vi "串口调试(hostlink).vi"(8 "error in (no error)":errorcluster caption="错误输入（无错误）", 11 "串口设置":T1={"VISA resource name"="COM1", "波特率"=9600, "数据位"=7, "停止位"=20, "奇偶位"=enum."Even"} {"停止位" items=["1.0"=10, "1.5"=15, "2.0"=20]; "数据位" items=["5"=5, "6"=6, "7"=7, "8"=8]; "波特率" items=["110"=110, "300"=300, "600"=600, "1200"=1200, "2400"=2400, "4800"=4800, "9600"=9600, "14400"=14400, "19200"=19200, "38400"=38400, "56000"=56000, "57600"=57600, "115200"=115200, "128000"=128000, "256000"=256000]}) -> (0 "error out":errorcluster caption="错误输出", 2 "串口状态":bool, 3 "串口初始化":T1)   [LabVIEW 2012]
uses:
  <vilib>/Instr/_visa.llb/VISA Flush IO Buffer Mask.ctl
  <vilib>/Instr/_visa.llb/VISA Configure Serial Port (Instr).vi
panel:
  out "返回码":string
  out "操作信息":string
  out "字符串接收区":string
  in  "过程停止按钮":bool
  in  "字符串发送区":string
  in  "发送":bool
  in  "取消按钮":bool
  in  "确定按钮":bool
  # "串口调试"
  # "(Omron Plc Hostlink 协议)"
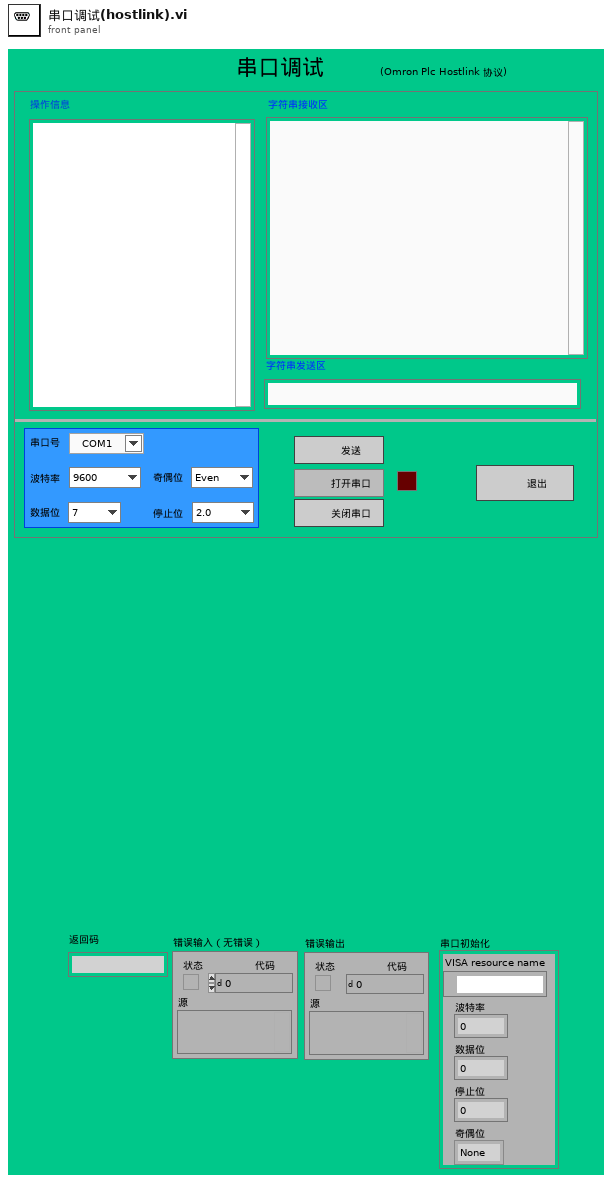
[diagram p1: front panel]
types:
  T1 = cluster{"VISA resource name":refnum<visa-resource-name>, "波特率":u32, "数据位":u16, "停止位":u16, "奇偶位":enum16{"None", "Odd", "Even", "Mark", "Space"}}
  T2 = typedef "VISA Flush IO Buffer Mask.ctl" = u16
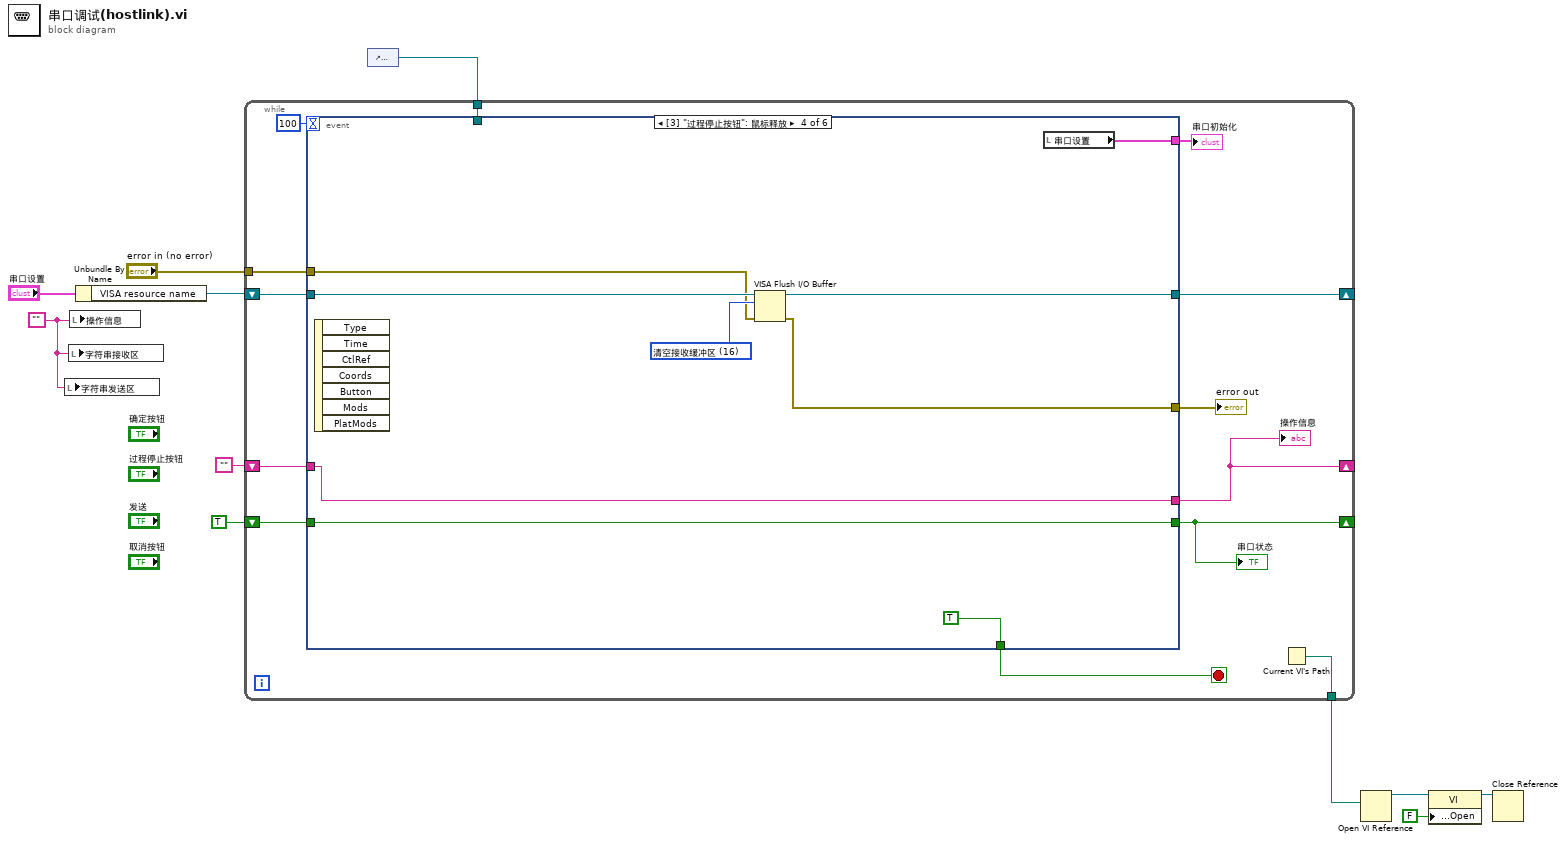
[diagram p0: block diagram]
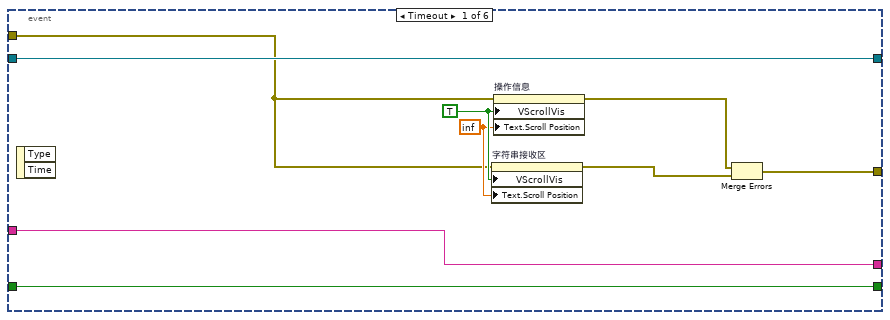
[diagram p2: hidden frame]
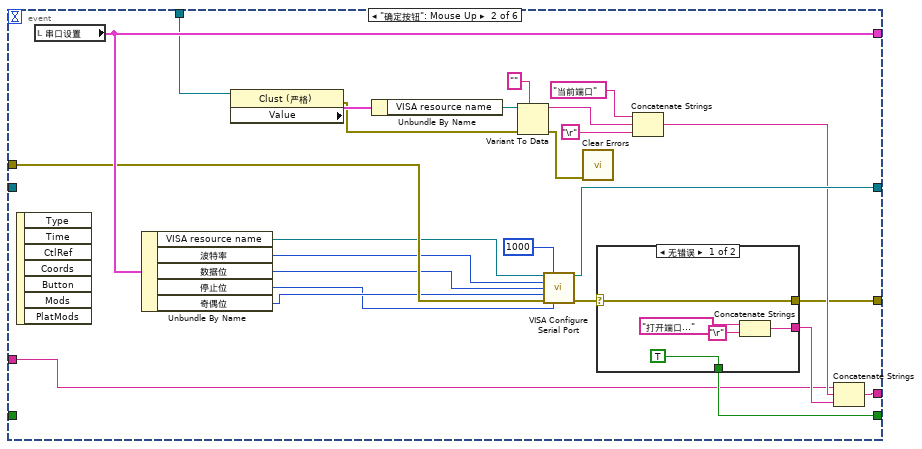
[diagram p3: hidden frame]
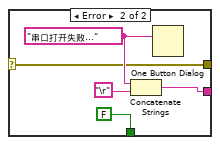
[diagram p4: hidden frame]
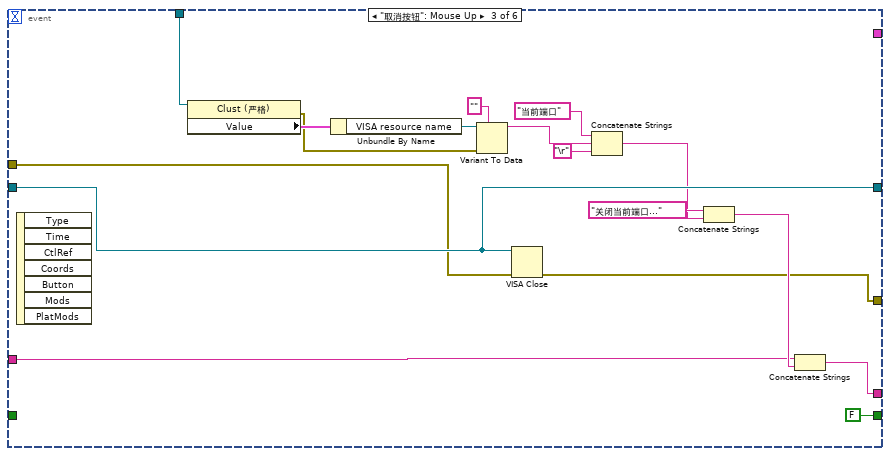
[diagram p5: hidden frame]
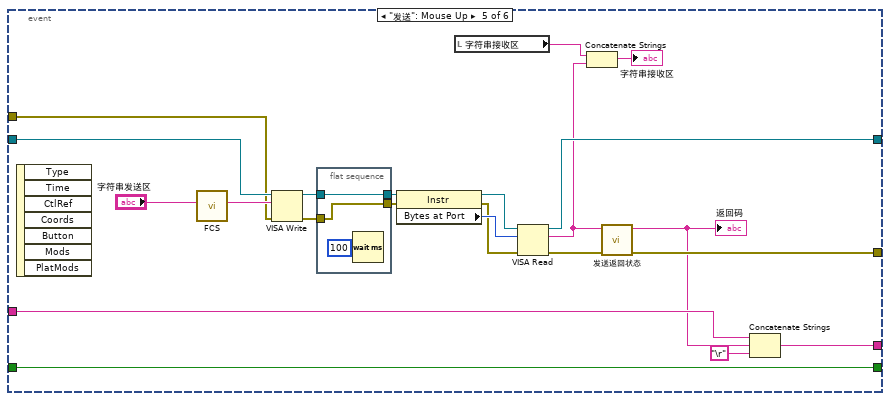
[diagram p6: hidden frame]
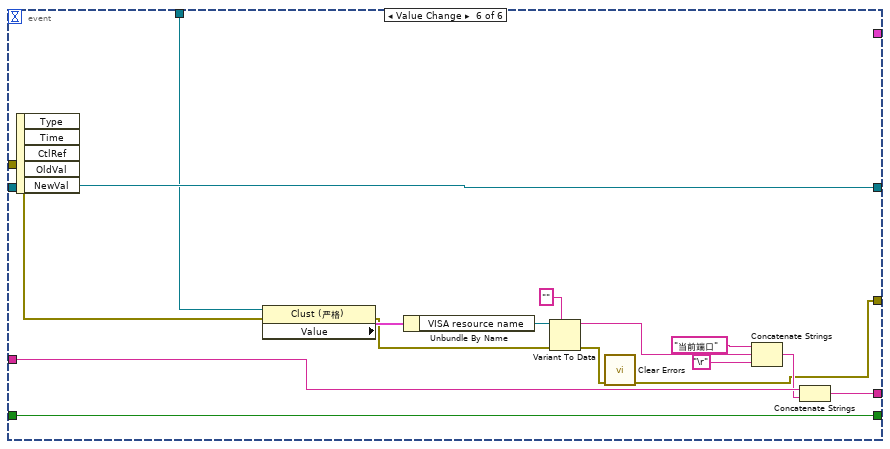
[diagram p7: hidden frame]
diagram:
  w5 = ""
  n1 = local write "字符串发送区"(w5) -> ()
  n2 = local write "字符串接收区"(w5) -> ()
  n3 = local write "操作信息"(w5) -> ()
  n4 = Unbundle By Name("串口设置") -> ("VISA resource name"=w11:refnum<visa-resource-name>)
  n5 = control-ref of="串口设置"() -> (w8:refnum<vi>)
  n6 = while {
    shift-right: [w24] -> _
    shift-left: w11 -> [w23]
    shift-right: [w13] -> _
    shift-left: TRUE -> [w20]
    shift-right: [w18] -> _
    shift-left: "" -> [w19]
    tunnel: w8 -> [w17]
    tunnel: "error in (no error)" -> [w16]
    tunnel: [w12] -> w1
    stop <- w22 stop-if-true
    n7 = event shown="[3] \"过程停止按钮\": 鼠标释放" {
      selector: _ -> [_ _ _ _ _ _]
      dyn-events: _ -> [_ _ _ _ _ _]
      timeout: 100 -> [_ _ _ _ _ _]
      tunnel: [w32 w57 FALSE w86 w99 w122] -> w13
      tunnel: [w33 w56 w84 w88 w113 w135] -> w24
      tunnel: w23 -> [w33 _ w84 w91 w116 _]
      tunnel: [_ _ _ TRUE _ _] -> w22
      tunnel: [_ w55 _ w92 _ _] -> w14
      tunnel: w20 -> [w32 _ _ w86 w99 w122]
      tunnel: w19 -> [w31 w45 w80 w93 w103 w128]
      tunnel: [w31 w46 w81 w93 w101 w126] -> w18
      tunnel: w17 -> [_ w42 w72 _ _ w123]
      tunnel: [w25 w41 w69 w87 w104 w121] -> w15
      tunnel: w16 -> [w28 w40 w70 w89 w106 w120]
      event Timeout {
        w29 = inf
        w30 = TRUE ("垂直滚动条可见")
        n8 = event-data() -> ()  [unwired: 1 in, 2 out]
        n9 = property on="字符串接收区" class="Str"(error in=w28, "VScrollVis"=w30, "Text.Scroll Position"=w29) -> (error out=w26:errorcluster)  [unwired: 1 in, 1 out]
        n10 = property on="操作信息" class="Str"(error in=w28, "VScrollVis"=w30, "Text.Scroll Position"=w29) -> (error out=w27:errorcluster)  [unwired: 1 in, 1 out]
        n11 = Merge Errors(w27, w26) -> (w25:errorcluster)
      }
      event "确定按钮": Mouse Up {
        n12 = event-data() -> ()  [unwired: 1 in, 7 out]
        n13 = local read "串口设置"() -> (w55:T1)
        n14 = Unbundle By Name(w55) -> ("VISA resource name"=w39:refnum<visa-resource-name>, "波特率"=w38:u32, "数据位"=w37:u16, "停止位"=w35:u16, "奇偶位"=w36:enum16{"None", "Odd", "Even", "Mark", "Space"})
        n15 = property class="Clust (严格)"(reference=w42) -> (error out=w44:errorcluster, "Value"=w54:T1)  [unwired: 1 in, 1 out]
        n16 = Unbundle By Name(w54) -> ("VISA resource name"=w53:refnum<visa-resource-name>)
        n17 = Variant To Data(error in=w44, type="", Variant=w53) -> (data=w50:string, error out=w43:errorcluster)
        n18 = call-poly "VISA Configure Serial Port"("VISA resource name"=w39, "timeout (10sec)"=u32 1000, "baud rate (9600)"=w38, "data bits (8)"=w37, "parity (0:none)"=w36, "error in (no error)"=w40, "stop bits (10: 1 bit)"=w35) -> ("VISA resource name out"=w56:refnum<visa-resource-name>, "error out"=w58:errorcluster)  [unwired: 7 in]
        n19 = call <vilib>:"Clear Errors.vi"("error in (no error)"=w43) -> ()  [unwired: 6 in, 1 out]
        n20 = case shown="无错误" w58 {
          selector: w58 -> [w59 w64]
          tunnel: [TRUE FALSE] -> w57
          tunnel: [w60 w65] -> w47
          tunnel: [w59 w64] -> w41
          frame No Error {
            n21 = Concatenate Strings("打开端口...", "\r") -> (w60:string)
          }
          frame Error {
            w66 = "串口打开失败..." ("消息")
            n22 = Concatenate Strings(w66, "\r") -> (w65:string)
            n23 = One Button Dialog(message=w66) -> ()  [unwired: 1 in, 1 out]
          }
        }
        n24 = Concatenate Strings("当前端口" ("字符串"), w50, "\r") -> (w48:string)
        n25 = Concatenate Strings(w45, w48, w47) -> (w46:string)
      }
      event "取消按钮": Mouse Up {
        n26 = event-data() -> ()  [unwired: 1 in, 7 out]
        n27 = property class="Clust (严格)"(reference=w72) -> (error out=w71:errorcluster, "Value"=w79:T1)  [unwired: 1 in, 1 out]
        n28 = Unbundle By Name(w79) -> ("VISA resource name"=w78:refnum<visa-resource-name>)
        n29 = Variant To Data(error in=w71, type="", Variant=w78) -> (data=w75:string)  [unwired: 1 out]
        n30 = VISA Close(VISA resource name=w84, error in (no error)=w70) -> (error out=w69:errorcluster)
        n31 = Concatenate Strings("当前端口" ("字符串"), w75, "\r") -> (w73:string)
        n32 = Concatenate Strings("关闭当前端口..." ("字符串"), w73) -> (w82:string)
        n33 = Concatenate Strings(w80, w82) -> (w81:string)
      }
      event "过程停止按钮": Mouse Up {
        w90 = T2 16 items=["清空接收缓冲区"=16, "向设备写入传输缓冲区"=32, "清空接收缓冲区（无I/O）"=64, "清空传输缓冲区"=128] ("Mask")
        n34 = event-data() -> ()  [unwired: 1 in, 7 out]
        n35 = VISA Flush I/O Buffer(VISA resource name=w91, mask (16)=w90, error in (no error)=w89) -> (VISA resource name out=w88:refnum<visa-resource-name>, error out=w87:errorcluster)
        n36 = local read "串口设置"() -> (w92:T1)
      }
      event "发送": Mouse Up {
        n37 = event-data() -> ()  [unwired: 1 in, 7 out]
        n38 = call "FCS.vi"("发送命令"="字符串发送区") -> ("完整帧"=w112:string)  [unwired: 10 in]
        n39 = VISA Write(VISA resource name=w116, write buffer=w112, error in (no error)=w106) -> (VISA resource name out=w111:refnum<visa-resource-name>, error out=w109:errorcluster)  [unwired: 1 out]
        n40 = flat-sequence {
          tunnel: w111 -> [w119]
          tunnel: [w119] -> w110
          tunnel: w109 -> [w118]
          tunnel: [w118] -> w108
          frame #0 {
            n41 = Wait (ms)(milliseconds to wait=100) -> ()  [unwired: 1 out]
          }
        }
        n42 = property class="Instr"(reference=w110, error in=w108) -> (reference out=w115:refnum<visa-resource-name>, error out=w107:errorcluster, "Bytes at Port"=w114:u32)
        n43 = local read "字符串接收区"() -> (w97:string)
        n44 = VISA Read(VISA resource name=w115, byte count=w114, error in (no error)=w107) -> (VISA resource name out=w113:refnum<visa-resource-name>, read buffer=w96:string, error out=w105:errorcluster)  [unwired: 1 out]
        n45 = Concatenate Strings(w97, w96) -> (→"字符串接收区":string)
        n46 = call "发送返回状态.vi"("错误输入"=w105, "字符串"=w96) -> ("错误输出"=w104:errorcluster, "返回"=w102:string)  [unwired: 8 in]
        "返回码" <- w102
        n47 = Concatenate Strings(w103, w102, "\r") -> (w101:string)
      }
      event "串口设置.VISA resource name": Value Change {
        n48 = event-data() -> ("NewVal"=w135:refnum<visa-resource-name>)  [unwired: 1 in, 4 out]
        n49 = property class="Clust (严格)"(reference=w123, error in=w120) -> (error out=w125:errorcluster, "Value"=w134:T1)  [unwired: 1 out]
        n50 = Unbundle By Name(w134) -> ("VISA resource name"=w133:refnum<visa-resource-name>)
        n51 = Variant To Data(error in=w125, type="", Variant=w133) -> (data=w130:string, error out=w124:errorcluster)
        n52 = call <vilib>:"Clear Errors.vi"("error in (no error)"=w124) -> ("error out"=w121:errorcluster)  [unwired: 6 in]
        n53 = Concatenate Strings("当前端口" ("字符串"), w130, "\r") -> (w127:string)
        n54 = Concatenate Strings(w128, w127) -> (w126:string)
      }
    }
    "操作信息" <- w18
    "error out" <- w15
    "串口初始化" <- w14
    "串口状态" <- w13
    n55 = Current VI's Path() -> (path=w12:path)
  }
  n56 = Open VI Reference(vi path=w1) -> (vi reference=w2:refnum<vi>)  [unwired: 5 in, 1 out]
  n57 = property on="Property Node" class="VI"(reference=w2, "Front Panel Window:Open"=FALSE ("前面板窗口:打开")) -> (reference out=w3:refnum<vi>)  [unwired: 1 in, 1 out]
  n58 = Close Reference(reference=w3) -> ()  [unwired: 1 in, 1 out]
